vi "Initialise.vi"(7 "PTI in":T1={"Delay before read (ms)"=0, "Mono 1"={"Timeout (ms)"=1000, "Resource Name"="COM1", "Baud Rate"=9600, "Data Bits"=8, "Parity"=0, "Stop Bits"=10, "Flow Control"=0}, "Mono 2"={"Timeout (ms)"=1000, "Resource Name"="COM1", "Baud Rate"=9600, "Data Bits"=8, "Parity"=0, "Stop Bits"=10, "Flow Control"=0}, "Two PTI Monochromators?"=FALSE} {"Mono 2"."Flow Control" items=["1.0"=10, "1.5"=15, "2.0"=20]; "Mono 2"."Stop Bits" items=["None", "Odd", "Even", "Mark", "Space"]; "Mono 2"."Parity" items=["None", "Odd", "Even", "Mark", "Space"]; "Mono 1"."Flow Control" items=["1.0"=10, "1.5"=15, "2.0"=20]; "Mono 1"."Stop Bits" items=["None", "Odd", "Even", "Mark", "Space"]; "Mono 1"."Parity" items=["None", "Odd", "Even", "Mark", "Space"]}, 8 "error in (no error)":errorcluster) -> (0 "error out":errorcluster, 5 "PTI out":T1={"Delay before read (ms)"=0, "Mono 1"={"Timeout (ms)"=1000, "Resource Name"="COM1", "Baud Rate"=9600, "Data Bits"=8, "Parity"=0, "Stop Bits"=10, "Flow Control"=0}, "Mono 2"={"Timeout (ms)"=1000, "Resource Name"="COM1", "Baud Rate"=9600, "Data Bits"=8, "Parity"=0, "Stop Bits"=10, "Flow Control"=0}, "Two PTI Monochromators?"=FALSE} {"Mono 2"."Flow Control" items=["1.0"=10, "1.5"=15, "2.0"=20]; "Mono 2"."Stop Bits" items=["None", "Odd", "Even", "Mark", "Space"]; "Mono 2"."Parity" items=["None", "Odd", "Even", "Mark", "Space"]; "Mono 1"."Flow Control" items=["1.0"=10, "1.5"=15, "2.0"=20]; "Mono 1"."Stop Bits" items=["None", "Odd", "Even", "Mark", "Space"]; "Mono 1"."Parity" items=["None", "Odd", "Even", "Mark", "Space"]})   [LabVIEW 2017, in "Monochromator.lvlib" / "PTI.lvlib"]
uses:
  PTI.lvlib
  Controls/Params.ctl
  Controls/VISA parameters.ctl
  Serial comms/Serial comms.lvlib
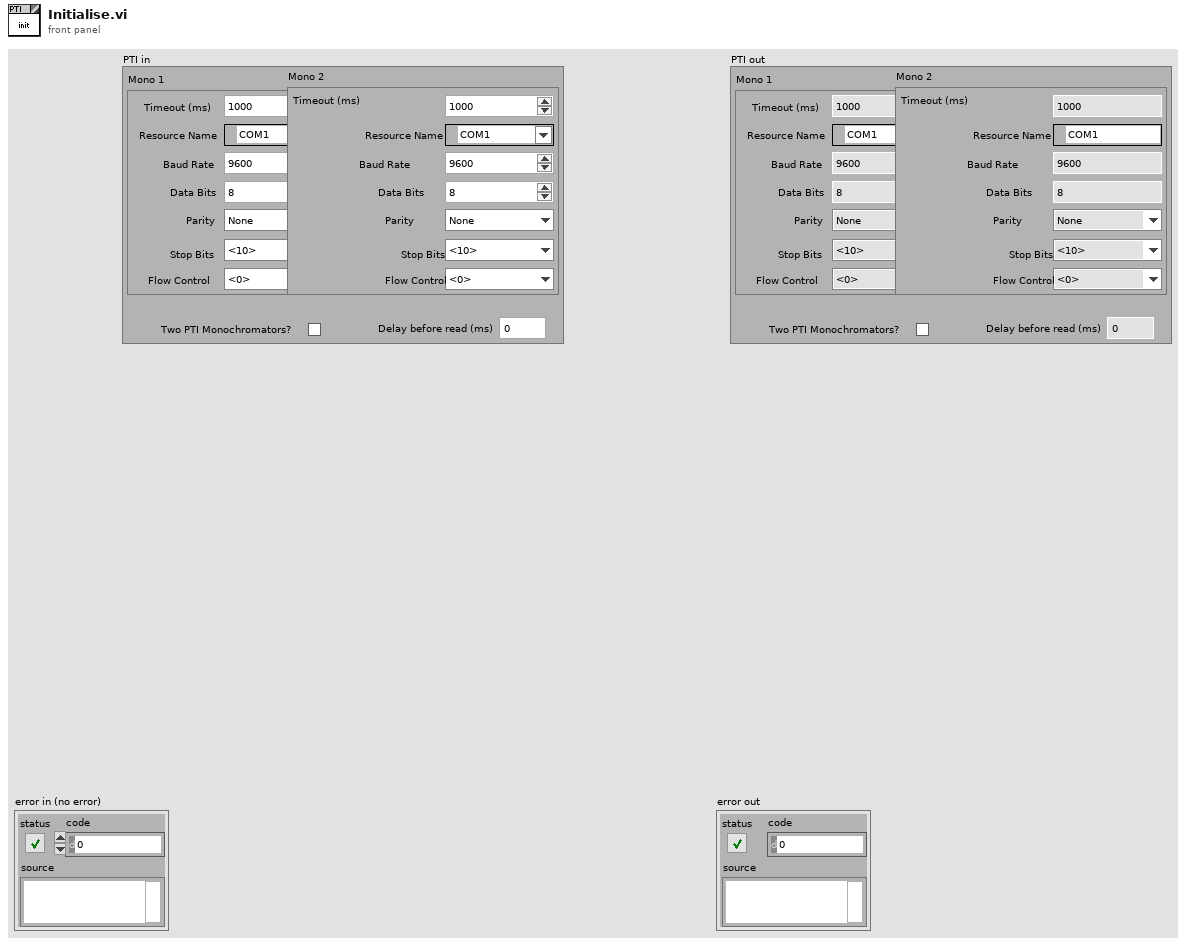
[diagram p1: front panel]
types:
  T1 = typedef "Monochromator.lvlib/PTI.lvlib/Params.ctl" = cluster{"Delay before read (ms)":u32, "Mono 1":T2, "Mono 2":T2, "Two PTI Monochromators?":bool}
  T2 = typedef "Serial comms.lvlib/VISA parameters.ctl" = cluster{"Timeout (ms)":u32, "Resource Name":refnum<visa-resource-name>, "Baud Rate":u32, "Data Bits":u16, "Parity":u16, "Stop Bits":u16, "Flow Control":u16}
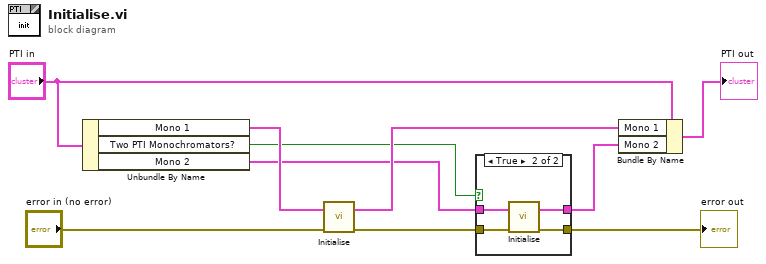
[diagram p0: block diagram]
diagram:
  n1 = Unbundle By Name("PTI in") -> ("Mono 1"=w8:T2, "Two PTI Monochromators?"=w1:bool, "Mono 2"=w3:T2)
  n2 = call "Initialise.vi"("VISA parameters"=w8, "error in"="error in (no error)") -> ("error out"=w10:errorcluster, "VISA parameters out"=w9:T2)  [unwired: 8 in]
  n3 = case shown="True" w1 {
    tunnel: w3 -> [w11 w16]
    tunnel: [w11 w15] -> w2
    tunnel: w10 -> [w12 w14]
    tunnel: [w12 w13] -> w5
    frame False {
    }
    frame True {
      n4 = call "Initialise.vi"("VISA parameters"=w16, "error in"=w14) -> ("error out"=w13:errorcluster, "VISA parameters out"=w15:T2)  [unwired: 8 in]
    }
  }
  "error out" <- w5
  n5 = Bundle By Name(cluster="PTI in", "Mono 1"=w9, "Mono 2"=w2) -> (→"PTI out":T1)
